vi "Multi line string to Array of Strings.vi"(6 "Multi Line String":string) -> (2 "Array of Strings":string[](array[string]))   [LabVIEW 2013]
doc: "Converts a multi line string into an array of strings. NOTE: This VI will remove any empty lines from the string!"
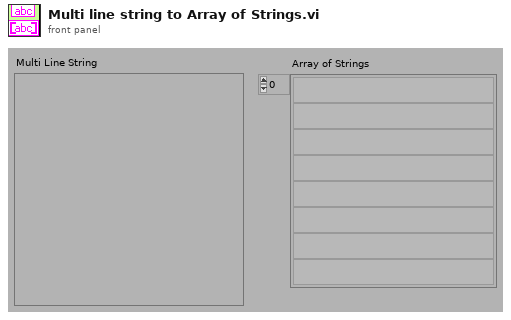
[diagram p1: front panel]
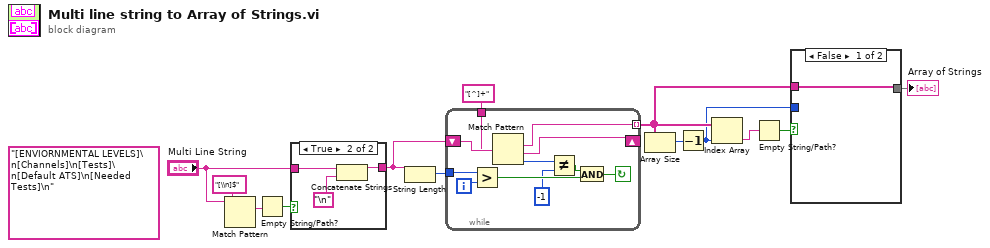
[diagram p0: block diagram]
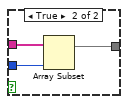
[diagram p2: hidden frame]
diagram:
  (unwired) "[ENVIORNMENTAL LEVELS]\n[Channels]\n[Tests]\n[Default ATS]\n[Needed Tests]\n"
  n1 = Match Pattern(string="Multi Line String", regular expression="[\\n]$") -> (match substring=w11:string)  [unwired: 4 out]
  n2 = Empty String/Path?(string/path=w11) -> (empty?=w10:bool)
  n3 = case shown="True" w10 {
    tunnel: "Multi Line String" -> [w14 w16]
    tunnel: [w14 w15] -> w9
    frame False {
    }
    frame True {
      n4 = Concatenate Strings(w16, "\n") -> (w15:string)
    }
  }
  n5 = String Length(string=w9) -> (length=w13:i32)
  n6 = while {
    tunnel: "[^]+" -> [w25]
    tunnel: [w23] -> w3 mode=indexing
    shift-left: w9 -> [w27]
    shift-right: [w24] -> _
    tunnel: w13 -> [w28]
    i -> [w26]
    stop <- w18 continue-if-true
    n7 = Greater?(x=w28, y=w26) -> (0:w22:bool)
    n8 = Match Pattern(string=w27, regular expression=w25) -> (match substring=w23:string, after substring=w24:string, offset past match=w21:i32)  [unwired: 2 out]
    n9 = Not Equal?(x=w21, y=-1) -> (x != y?=w19:bool)
    n10 = And(x=w19, y=w22) -> (x .and. y?=w18:bool)
  }
  n11 = Array Size(array=w3) -> (size(s)=w6:i32)
  n12 = Decrement(x=w6) -> (x-1=w2:i32)
  n13 = Index Array(array=w3, index=w2) -> (element=w5:string)
  n14 = Empty String/Path?(string/path=w5) -> (empty?=w4:bool)
  n15 = case shown="False" w4 {
    tunnel: w3 -> [w29 w32]
    tunnel: w2 -> [_ w31]
    tunnel: [w29 w30] -> w1
    frame False {
    }
    frame True {
      n16 = Array Subset(array=w32, length=w31) -> (w30:string[])  [unwired: 1 in]
    }
  }
  "Array of Strings" <- w1
